vi "SE_E5_Práctica4.vi"() -> ()   [LabVIEW 2015]
panel:
  in  "Boolean 2":bool
  in  "Boolean":bool
  out "Waveform Chart":dbl[](graph)
  in  "stop":bool
  out "Instantaneo":dbl(graph)
  out "Thermometer":dbl(slide) scale=-200.0..360.0
  in  "Slide":dbl(slide) scale=0.0..350.0
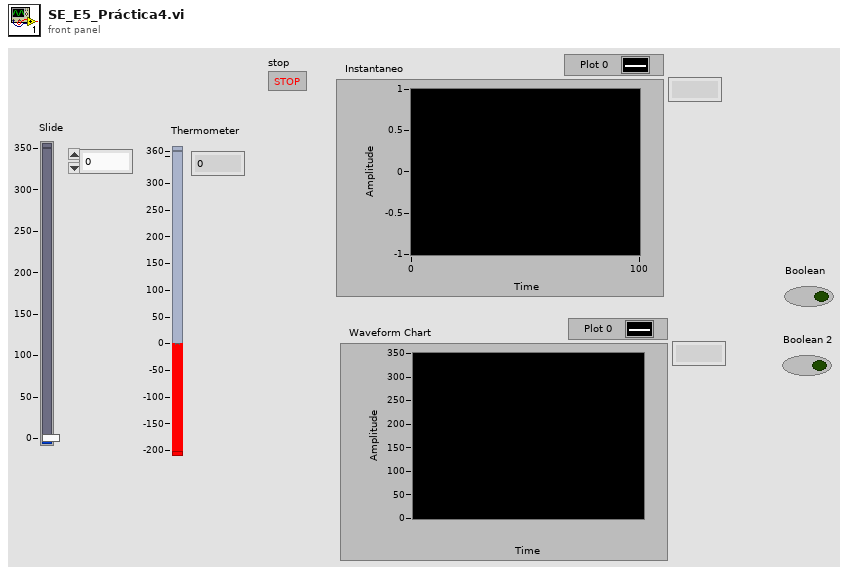
[diagram p1: front panel]
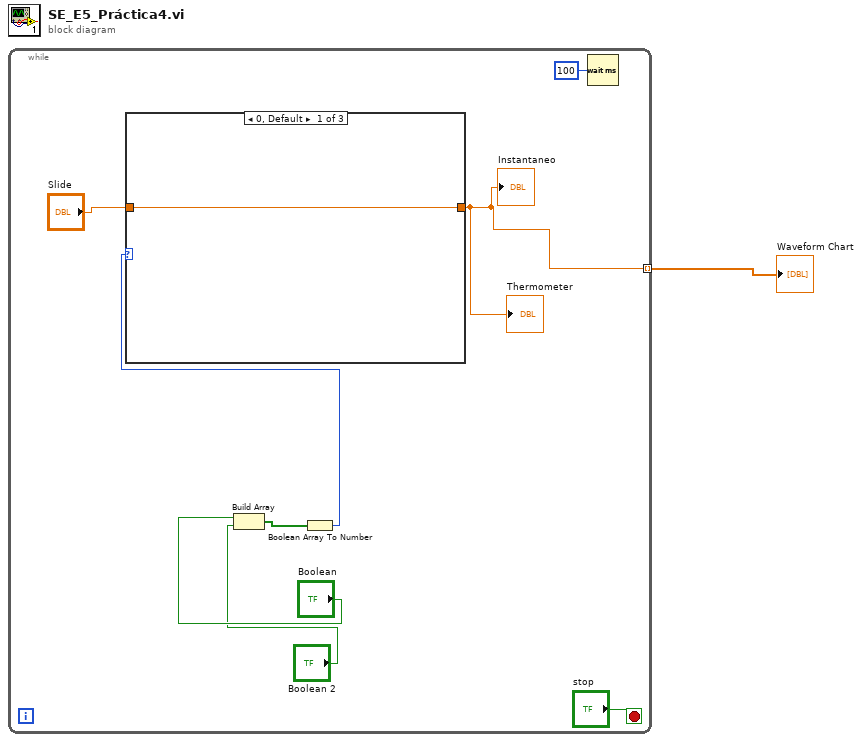
[diagram p0: block diagram]
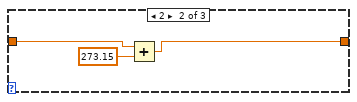
[diagram p2: hidden frame]
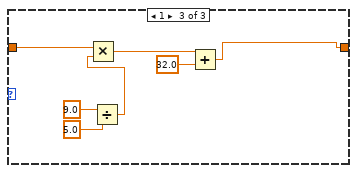
[diagram p3: hidden frame]
diagram:
  n1 = while {
    tunnel: [w5] -> w1 mode=indexing
    stop <- "stop" stop-if-true
    n2 = Build Array("Boolean", "Boolean 2") -> (w7:bool[])
    n3 = Boolean Array To Number(Boolean array=w7) -> (number=w6:u32)
    n4 = case shown="0, Default" w6 {
      tunnel: "Slide" -> [w10 w11 w20]
      tunnel: [w10 w12 w15] -> w5
      frame 0, Default {
      }
      frame 2 {
        n5 = Add(x=w11, y=273.15) -> (x+y=w12:dbl)
      }
      frame 1 {
        n6 = Divide(x=9.0, y=5.0) -> (x/y=w19:dbl)
        n7 = Multiply(x=w20, y=w19) -> (x*y=w16:dbl)
        n8 = Add(x=w16, y=32.0) -> (x+y=w15:dbl)
      }
    }
    "Thermometer" <- w5
    "Instantaneo" <- w5
    n9 = Wait (ms)(milliseconds to wait=u32 100) -> ()  [unwired: 1 out]
  }
  "Waveform Chart" <- w1
